vi "Run Spectrogram.vi"(9 "Channel Name":string, 10 "Signal":waveform(dbl)={"t0"=timestamp(0 s since 1904-01-01), "dt"=0.0, "Y"=[]}, 11 "Data in":T1={"First Time"=FALSE, "Show Spectrogram Window"=TRUE, "Show Spectrogram Window Button Clicked"=FALSE, "Extension"=0, "Time steps"=-1, "Frequency bins"=512, "Type"=1, "Length"=-1, "Color Table"=0, "Spectrogram VI Ref"=refnum} {"Color Table" items=["Rainbow", "Inverse gray", "Gray", "Color table 1", "Color table 2", "Color table 3"]; "Type" items=["None ", "Hanning", "Hamming", "Blackman-Harris", "Exact Blackman", "Blackman", "Flat Top", "4 Term B-Harris ", "7 Term B-Harris", "Low Sidelobe", "Gaussian"]; "Extension" items=["Zero padding", "Symmetric", "Periodic"]}) -> (3 "Data out":T1={"First Time"=FALSE, "Show Spectrogram Window"=TRUE, "Show Spectrogram Window Button Clicked"=FALSE, "Extension"=0, "Time steps"=-1, "Frequency bins"=512, "Type"=1, "Length"=-1, "Color Table"=0, "Spectrogram VI Ref"=refnum} {"Color Table" items=["Rainbow", "Inverse gray", "Gray", "Color table 1", "Color table 2", "Color table 3"]; "Type" items=["None ", "Hanning", "Hamming", "Blackman-Harris", "Exact Blackman", "Blackman", "Flat Top", "4 Term B-Harris ", "7 Term B-Harris", "Low Sidelobe", "Gaussian"]; "Extension" items=["Zero padding", "Symmetric", "Periodic"]})   [LabVIEW 2023, in "Spectrogram.lvlib" / "Spectrogram.lvclass"]
uses:
  Spectrogram.lvclass
  Spectrogram Data.ctl
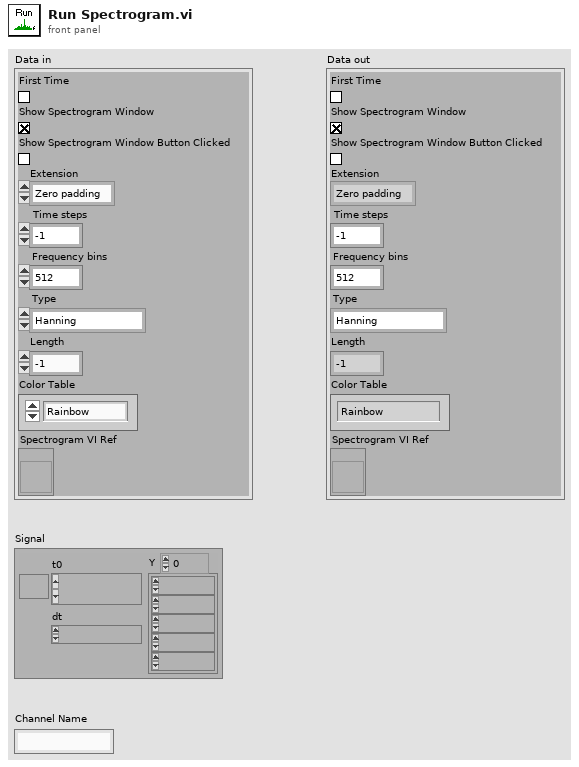
[diagram p1: front panel]
types:
  T1 = typedef "Spectrogram.lvlib/Spectrogram.lvclass/Spectrogram Data.ctl" = cluster{"First Time":bool, "Show Spectrogram Window":bool, "Show Spectrogram Window Button Clicked":bool, "Extension":u16, "Time steps":i32, "Frequency bins":i32, "Type":i32, "Length":i32, "Color Table":u16, "Spectrogram VI Ref":refnum<vi>}
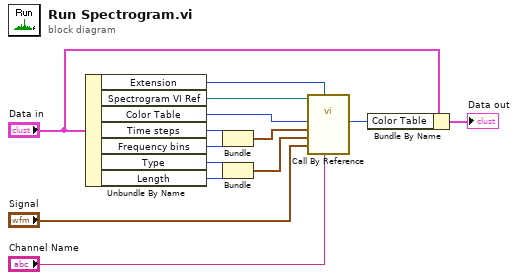
[diagram p0: block diagram]
diagram:
  n1 = Unbundle By Name("Data in") -> ("Extension"=w11:u16, "Spectrogram VI Ref"=w12:refnum<vi>, "Color Table"=w10:u16, "Time steps"=w9:i32, "Frequency bins"=w8:i32, "Type"=w7:i32, "Length"=w6:i32)
  n2 = Bundle("Time steps"=w9, "Frequency bins"=w8) -> (w5:cluster{"Time steps":i32, "Frequency bins":i32})  [unwired: 1 in]
  n3 = Bundle("Type"=w7, "Length"=w6) -> (w4:cluster{"Type":i32, "Length":i32})  [unwired: 1 in]
  n4 = call-by-ref "?"(reference=w12, "Channel Name"="Channel Name", "Extension"=w11, "Signal"="Signal", "Window"=w4, "Time-frequency sampling"=w5, "Color Table in"=w10) -> ("Color Table out"=w3:u16)  [unwired: 6 in, 2 out]
  n5 = Bundle By Name(cluster="Data in", "Color Table"=w3) -> (→"Data out":T1)
